vi "DWDT Digital Size.vi"(8 "error in (no error)":errorcluster caption="错误输入（无错误）", 11 "digital waveform in":digitalwaveform(waveform)={"t0"=timestamp(0 s since 1904-01-01), "dt"=0.0, "Y"={"transitions"=[], "data"=[]}, "error"={"status"=FALSE, "code"=37421928, "source"=""}} caption="数字波形输入") -> (0 "error out":errorcluster caption="错误输出", 1 "number of signals":i32 caption="信号数", 2 "number of samples":i32 caption="采样数", 3 "digital waveform out":digitalwaveform(waveform)={"t0"=timestamp(0 s since 1904-01-01), "dt"=0.0, "Y"={"transitions"=[], "data"=[]}, "error"={"status"=FALSE, "code"=37421928, "source"=""}} caption="数字波形输出")   [LabVIEW 2018]
doc: "返回数字输入中包含的采样和信号的数量。 通过连线数据至<B>数字波形输入</B>输入端可确定要使用的多态实例，也可手动选择实例。"
panel:
  in  "Empty Digital Waveform":digitalwaveform(waveform)={"t0"=timestamp(0 s since 1904-01-01), "dt"=0.0, "Y"={"transitions"=[], "data"=[]}, "error"={"status"=FALSE, "code"=37421928, "source"=""}} caption="空数字波形"
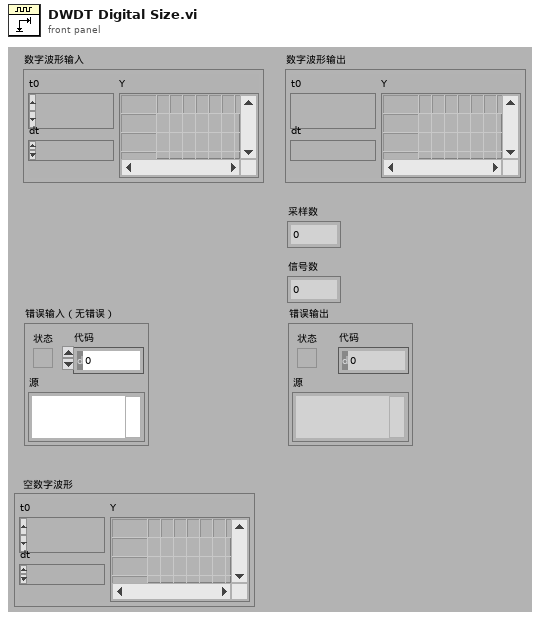
[diagram p1: front panel]
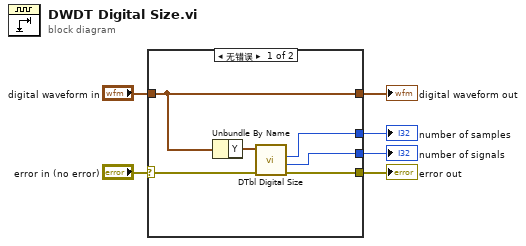
[diagram p0: block diagram]
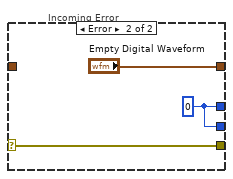
[diagram p2: hidden frame]
diagram:
  n1 = case shown="无错误" "error in (no error)" {
    selector: "error in (no error)" -> [w10 w15]
    tunnel: "digital waveform in" -> [w8 _]
    tunnel: [w8 "Empty Digital Waveform"] -> w5
    tunnel: [w11 w14] -> w6
    tunnel: [w9 w15] -> w3
    tunnel: [w12 w14] -> w1
    frame No Error {
      n2 = Unbundle By Name(w8) -> ("Y"=w7:digitaldata)
      n3 = call "DTbl Digital Size.vi"("error in (no error)"=w10, "digital data in"=w7) -> ("error out"=w9:errorcluster, "number of signals"=w11:i32, "number of samples"=w12:i32)  [unwired: 6 in, 1 out]
    }
    frame Error {
      w14 = 0
      # "Incoming Error"
    }
  }
  "number of signals" <- w6
  "digital waveform out" <- w5
  "error out" <- w3
  "number of samples" <- w1
